vi "BME_DG_ReadTriggerCounter64Bit.vi"(8 "error in (no error)":errorcluster, 11 "DG_Number":i32) -> (0 "error out":errorcluster, 3 "Counter":i64)   [LabVIEW 2009, in "POLARIS BME DG.lvlib"]
uses:
  POLARIS BME DG.lvlib
  BME DLL/DelayGenerator.dll
panel:
  in  "tmp":i64
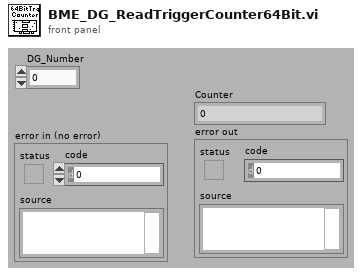
[diagram p1: front panel]
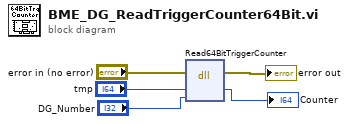
[diagram p0: block diagram]
diagram:
  n1 = dll-call lib="C:/CS Framework/LVSCC/LV2009/GPL/Projects/cs-framework/CSClass/CSPOLARIS/POLARIS BME DG/BME DLL/DelayGenerator.dll" fn="Read64BitTriggerCounter" label="Read_DG_Status"(error in="error in (no error)", "Counter"="tmp", "DG_Number"="DG_Number") -> (error out=→"error out":errorcluster, "Counter"=→"Counter":i64)  [unwired: 4 in, 1 out]
